vi "Measure-Z.vi"(7 "QuWire in":refnum<class "QuWire.lvclass">) -> (8 "QuWire out":refnum<class "QuWire.lvclass">, 15 "Classical bit":bool)   [LabVIEW 2020]
doc: "Measure Qubit (Z-Basis)\n\nPerforms a projective measurement.\n\n1. Calculates probability of |0> vs |1>.\n2. Collapses state vector to the result.\n3. Renormalizes the state."
uses:
  QuSim/QuWire/QuWire.lvclass
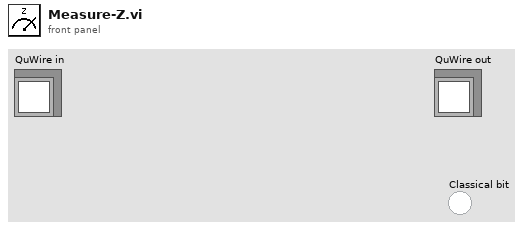
[diagram p1: front panel]
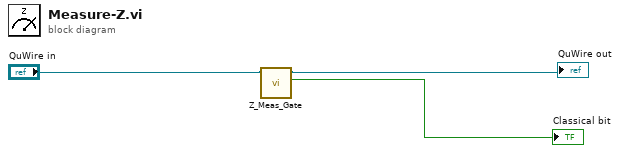
[diagram p0: block diagram]
diagram:
  n1 = call "Z_Meas_Gate.vi"("QuWire in"="QuWire in") -> ("Classical bit"=→"Classical bit":bool, "QuWire out"=→"QuWire out":refnum<class "QuWire.lvclass">)  [unwired: 8 in, 1 out]
